vi "Export_Add Device.vi"(11 "Export Setting in":T1) -> (3 "Export Setting out":T1)   [LabVIEW 2015, in "ConfigHelper.lvlib"]
uses:
  ConfigHelper.lvlib
  Control_UI_Export Setting.ctl
  Control_UI_Export Setting State.ctl
  <vilib>/addons/PointValueMap/controls/PointMap.ctl
  Control_Export File Setup.ctl
  Control_Export Setup.ctl
  <vilib>/addons/PointValueMap/PointValueMap.lvlib
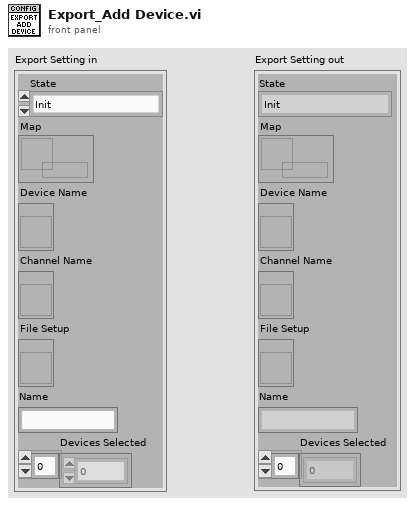
[diagram p1: front panel]
types:
  T1 = typedef "ConfigHelper.lvlib/Control_UI_Export Setting.ctl" = cluster{"State":T2, "Map":T3, "Device Name":refnum<vi>, "Channel Name":refnum<vi>, "File Setup":refnum<vi>, "Name":string, "Devices Selected":i32[]}
  T2 = typedef "ConfigHelper.lvlib/Control_UI_Export Setting State.ctl" = enum16{"Init", "Wait", "Exit", "Write to File", "Read from PVM", "Write to PVM", "Update Device", "Add Device", "Remove Device", "Copy Device", "Update Channel", "Add Channel", "Remove Channel", "Import from TDMS"}
  T3 = typedef "PointValueMap.lvlib/PointMap.ctl" = refnum<data-value>
  T4 = enum8{"Enabled", "Disabled", "Disabled and Grayed Out"}
  T5 = typedef "ConfigHelper.lvlib/Control_Export File Setup.ctl" = cluster{"CSV":bool, "TDMS":bool, "RAW TDMS":bool}
  T6 = typedef "ConfigHelper.lvlib/Control_Export Setup.ctl" = cluster{"Device Name":string, "Export CSV":bool, "Export TDMS":bool, "Export RAW TDMS":bool, "Channel Names":string[]}
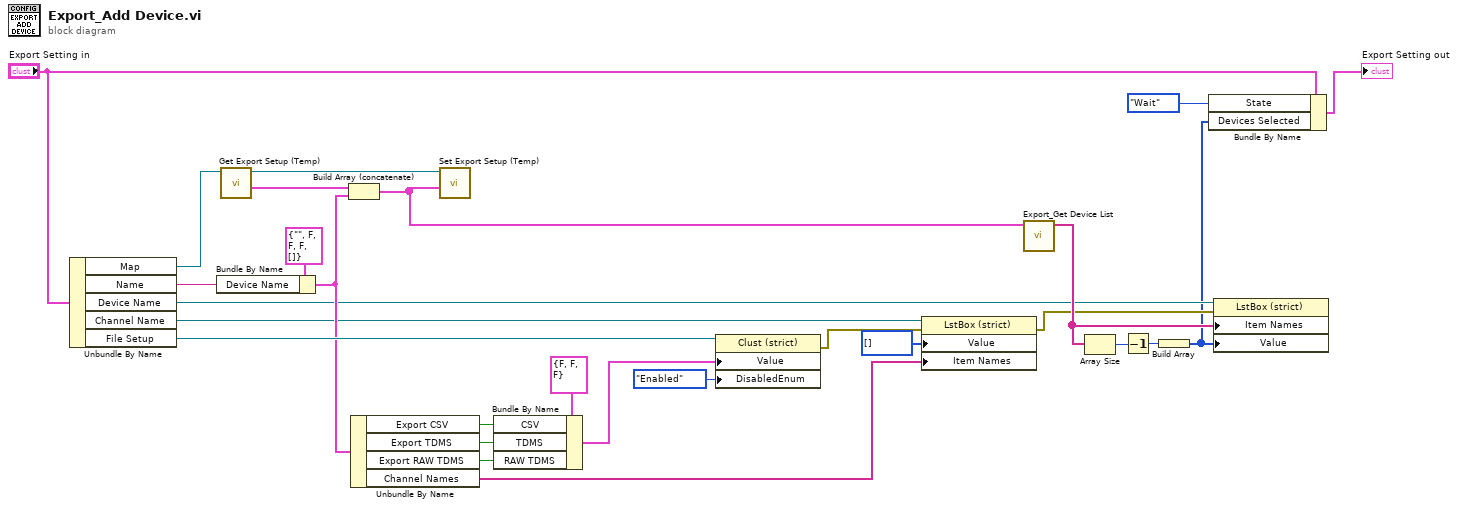
[diagram p0: block diagram]
diagram:
  n1 = Unbundle By Name("Export Setting in") -> ("Map"=w24:T3, "Name"=w22:string, "Device Name"=w7:refnum<vi>, "Channel Name"=w10:refnum<vi>, "File Setup"=w17:refnum<vi>)
  n2 = Bundle By Name(cluster=T6 {"Device Name"="", "Export CSV"=FALSE, "Export TDMS"=FALSE, "Export RAW TDMS"=FALSE, "Channel Names"=[]} ("Device Export Setup"), "Device Name"=w22) -> (w16:T6)
  n3 = call "Get Export Setup (Temp).vi"("Map"=w24) -> ("Export Setup"=w21:T6[], "Map Out"=w20:T3)  [unwired: 8 in, 1 out]
  n4 = Build Array (concatenate)(w21, w16) -> (w19:T6[])
  n5 = Unbundle By Name(w16) -> ("Export CSV"=w14:bool, "Export TDMS"=w13:bool, "Export RAW TDMS"=w12:bool, "Channel Names"=w9:string[])
  n6 = call "Set Export Setup (Temp).vi"("Export Setup"=w19, "Map"=w20) -> ()  [unwired: 8 in, 2 out]
  n7 = Bundle By Name(cluster=T5 {"CSV"=FALSE, "TDMS"=FALSE, "RAW TDMS"=FALSE} ("Export File Setup"), "CSV"=w14, "TDMS"=w13, "RAW TDMS"=w12) -> (w11:T5)
  n8 = property class="Clust (strict)"(reference=w17, "Value"=w11, "DisabledEnum"=T4."Enabled" ("Disabled")) -> (error out=w5:errorcluster)  [unwired: 1 in, 1 out]
  n9 = property class="LstBox (strict)"(reference=w10, error in=w5, "Value"=i32[] [], "Item Names"=w9) -> (error out=w6:errorcluster)  [unwired: 1 out]
  n10 = call "Export_Get Device List.vi"("Export Setting"=w19) -> ("Device Names"=w18:string[])  [unwired: 10 in]
  n11 = Array Size(array=w18) -> (size(s)=w2:i32)
  n12 = Decrement(x=w2) -> (x-1=w3:i32)
  n13 = Build Array(w3) -> (w1:i32[])
  n14 = Bundle By Name(cluster="Export Setting in", "State"=Control_UI_Export_Setting_State."Wait", "Devices Selected"=w1) -> (→"Export Setting out":T1)
  n15 = property class="LstBox (strict)"(reference=w7, error in=w6, "Item Names"=w18, "Value"=w1) -> ()  [unwired: 2 out]
